vi "H5Fcreate.vi"(4 "access_id":T1, 5 "create_id":T1, 6 "error in (no error)":errorcluster, 7 "flags":u32(ring)=2 items=["H5F_ACC_TRUNC"=2, "H5F_ACC_EXCL"=4], 9 "path":path) -> (0 "error out":errorcluster, 3 "HDF5 Ref":T1)   [LabVIEW 2017]
doc: "Creates an HDF5 file."
uses:
  <vilib>/UPVI/lvhdf5/library.llb/HDF5 Ref.ctl
  <vilib>/UPVI/lvhdf5/hdf5.dll
panel:
  # "LVHDF5 Toolkit\nCopyright (c) 2005-2013 by Jason D. Sommerville\nCopyright (c) 2014 by UPVI, LLC.\n\nThis use and distribution of this file is governed by the terms found in \nLICENSE.txt distributed with this toolkit and installed at\n <user.lib>\\_lvhdf5\\LICENSE.txt"
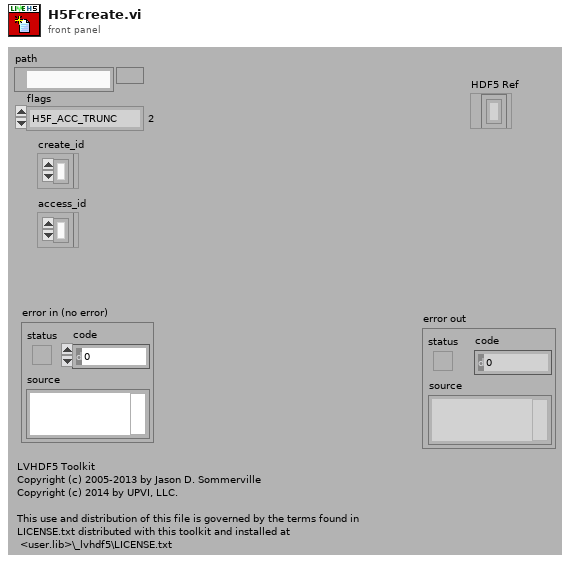
[diagram p1: front panel]
types:
  T1 = typedef "HDF5 Ref.ctl" = refnum<k1>
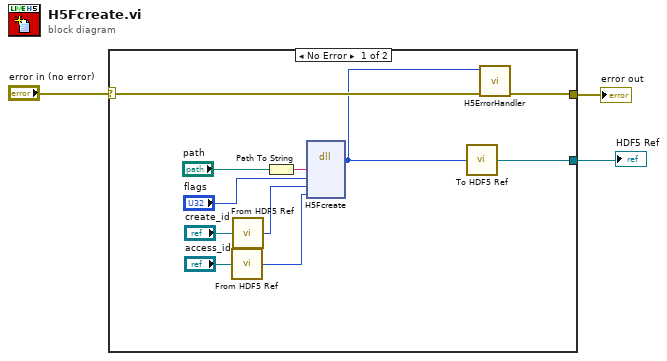
[diagram p0: block diagram]
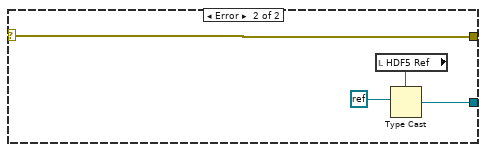
[diagram p2: hidden frame]
diagram:
  n1 = case shown="No Error" "error in (no error)" {
    selector: "error in (no error)" -> [w14 w18]
    tunnel: [w13 w18] -> w2
    tunnel: [w9 w15] -> w1
    frame No Error {
      n2 = call <vilib>:"From HDF5 Ref.vi"("HDF5 Ref"="access_id") -> ("I32"=w4:i32)
      n3 = call <vilib>:"From HDF5 Ref.vi"("HDF5 Ref"="create_id") -> ("I32"=w6:i32)
      n4 = Path To String(path="path") -> (string=w12:string)
      n5 = dll-call lib="C:/Program Files/National Instruments/LabVIEW 2017/vi.lib/UPVI/lvhdf5/hdf5.dll" fn="H5Fcreate"("file_path"=w12, "flags"="flags", "create_id"=w6, "access_id"=w4) -> ("return type"=w8:i32)  [unwired: 7 in, 2 out]
      n6 = call <vilib>:"To HDF5 Ref.vi"("I32"=w8) -> ("HDF5 Ref"=w9:T1)
      n7 = call <vilib>:"H5ErrorHandler.vi"("error in (no error)"=w14, "herr_t"=w8) -> ("error out"=w13:errorcluster)  [unwired: 3 in, 4 out]
    }
    frame Error {
      n8 = local read "HDF5 Ref"() -> (w17:T1)
      n9 = Type Cast(type=w17, x=refnum<k0> refnum) -> (*(type *) &x=w15:T1)
    }
  }
  "error out" <- w2
  "HDF5 Ref" <- w1
